vi "single cycle kalman step.vi"(0 "state in":T1, 1 "apply measurement":bool, 5 "location":T4, 9 "pixel values cluster":T3, 11 "feedback channel":enum16{"channel 0", "channel 1", "both"}(ring)=enum."both", 12 "half valid z-range (ncycles * 64)":i16=500, 13 "Vz feedback?":bool) -> (4 "state out":T1)   [LabVIEW 2010]
uses:
  kalman 3-axis state.ctl
  integrating single axis kalman state.ctl
  common_typedefs/channels_cluster.ctl
panel:
  # "1 z-level = 3.4*10^-4 * scan amplitude\nat A = 30 um, 1 z-level = 10 nm"
  # "full scan range -> half valid z > 9143 (=143 * 64)"
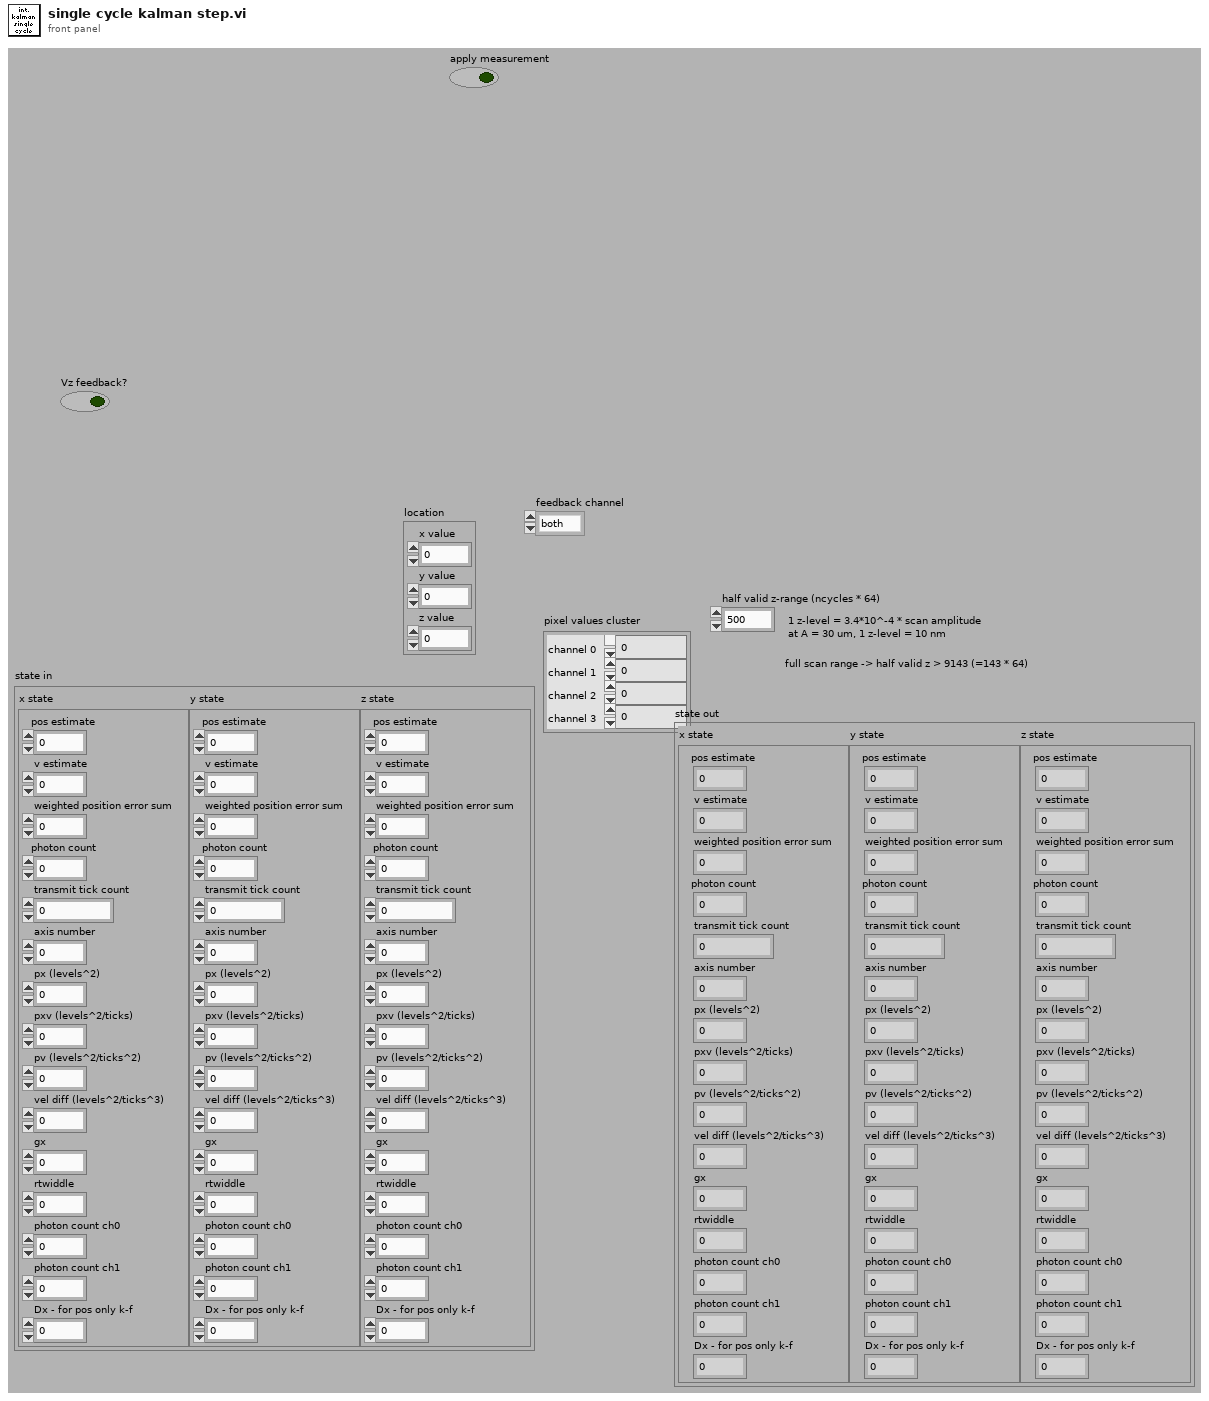
[diagram p1: front panel]
types:
  T1 = typedef "kalman 3-axis state.ctl" = cluster{"x state":T2, "y state":T2, "z state":T2}
  T2 = typedef "integrating single axis kalman state.ctl" = cluster{"pos estimate":fxp<+/-,32,16>, "v estimate":fxp<+/-,16,0>, "weighted position error sum":fxp<+/-,32,32>, "photon count":u32, "transmit tick count":u32, "axis number":u8, "px (levels^2)":fxp<+,32,19>, "pxv (levels^2/ticks)":fxp<+,32,2>, "pv (levels^2/ticks^2)":fxp<+,32,-14>, "vel diff (levels^2/ticks^3)":fxp<+,24,-22>, "gx":fxp<+,16,8>, "rtwiddle":fxp<+,16,26>, "photon count ch0":u32, "photon count ch1":u32, "Dx - for pos only k-f":fxp<+,32,19>}
  T3 = typedef "channels_cluster.ctl" = cluster{"channel 0":u32, "channel 1":u32, "channel 2":u32, "channel 3":u32}
  T4 = cluster{"x value":i16, "y value":i16, "z value":i16}
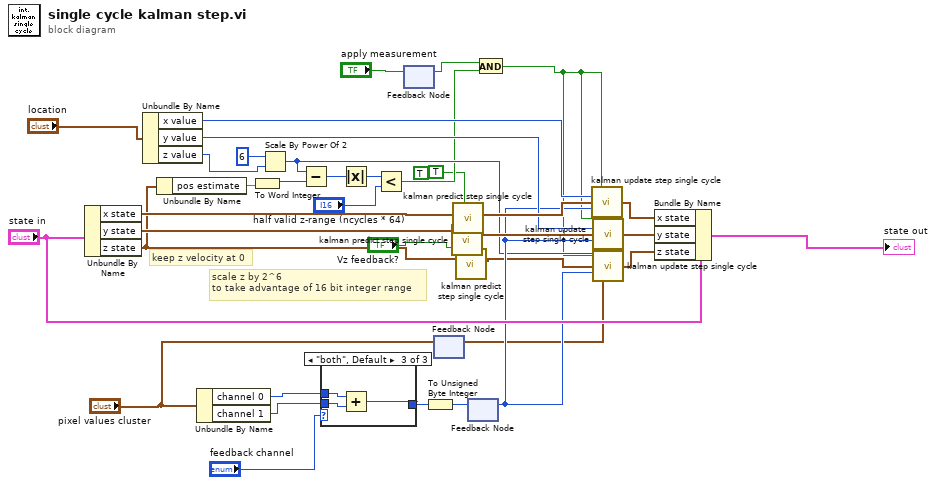
[diagram p0: block diagram]
diagram:
  # "keep z velocity at 0"
  # "scale z by 2^6\nto take advantage of 16 bit integer range"
  n1 = Unbundle By Name("state in") -> ("x state"=w37:T2, "y state"=w36:T2, "z state"=w15:T2)
  n2 = Unbundle By Name("location") -> ("x value"=w35:i16, "y value"=w32:i16, "z value"=w13:i16)
  n3 = Unbundle By Name(w15) -> ("pos estimate"=w14:fxp<+/-,32,16>)
  n4 = Unbundle By Name("pixel values cluster") -> ("channel 0"=w26:u32, "channel 1"=w25:u32)
  n5 = To Word Integer(number=w14) -> (16bit integer=w12:i16)
  n6 = Scale By Power Of 2(n=6, x=w13) -> (x*2^n=w8:i16)
  n7 = Subtract(x=w8, y=w12) -> (x-y=w11:i16)
  n8 = case shown="\"both\", Default" "feedback channel" {
    tunnel: w26 -> [w38 _ w42]
    tunnel: w25 -> [_ w39 w41]
    tunnel: [w38 w39 w40] -> w22
    frame "channel 0" {
    }
    frame "channel 1" {
    }
    frame "both", Default {
      n9 = Add(x=w42, y=w41) -> (x+y=w40:u32)
    }
  }
  n10 = Absolute Value(x=w11) -> (abs(x)=w10:i16)
  n11 = Less?(x=w10, y="half valid z-range (ncycles * 64)") -> (x < y?=w5:bool)
  n12 = feedback-in #1("apply measurement") -> ()
  n13 = feedback #1() -> (w4:bool)  [unwired: 1 in]
  n14 = To Unsigned Byte Integer(number=w22) -> (unsigned 8bit integer=w21:u8)
  n15 = feedback-in #2("pixel values cluster") -> ()
  n16 = feedback #2() -> (w16:T3)  [unwired: 1 in]
  n17 = call "kalman predict step single cycle.vi"("v-feedback"=TRUE, "state in"=w36) -> ("state out"=w33:T2)  [unwired: 9 in]
  n18 = call "kalman predict step single cycle.vi"("v-feedback"=TRUE, "state in"=w37) -> ("state out"=w34:T2)  [unwired: 9 in]
  n19 = call "kalman predict step single cycle.vi"("v-feedback"="Vz feedback?", "state in"=w15) -> ("state out"=w18:T2)  [unwired: 9 in]
  n20 = feedback-in #3(w21) -> ()
  n21 = feedback #3() -> (w20:u8)  [unwired: 1 in]
  n22 = And(x=w4, y=w5) -> (x .and. y?=w6:bool)
  n23 = call "kalman update step single cycle.vi"("apply measurement?"=w6, "location"=w35, "state in"=w34, "num photons"=w20, "pixel values cluster"=w16) -> ("state out"=w30:T2)  [unwired: 10 in]
  n24 = call "kalman update step single cycle.vi"("apply measurement?"=w6, "location"=w32, "state in"=w33, "num photons"=w20, "pixel values cluster"=w16) -> ("state out"=w29:T2)  [unwired: 10 in]
  n25 = call "kalman update step single cycle.vi"("apply measurement?"=w6, "location"=w8, "state in"=w18, "num photons"=w20, "pixel values cluster"=w16) -> ("state out"=w28:T2)  [unwired: 10 in]
  n26 = Bundle By Name(cluster="state in", "x state"=w30, "y state"=w29, "z state"=w28) -> (→"state out":T1)
